vi "Save_to_Project.vi"(8 "error in (no error)":errorcluster, 9 "index":string, 10 "buildObject":T1, 11 "Class in":refnum<class "IB_DistPart.lvclass">) -> (0 "error out":errorcluster, 2 "buildObject out":T1, 3 "Class out":refnum<class "IB_DistPart.lvclass">, 5 "saved?":bool)   [LabVIEW 2020, in "IB_DistPart.lvclass"]
uses:
  <vilib>/AppBuilder/IB_Classes/DistPart/IB_DistPart.lvclass
  <vilib>/AppBuilder/IB_Classes/DistPart/IB_DistPart.lvclass/IB_DistPart.ctl
  <vilib>/AppBuilder/IB_RW_Project/IB_RW_Project_PropBag_Action.ctl
  <vilib>/AppBuilder/IB_Classes/SoftDependency/IB_SoftDependency.lvclass
  <resource>/Framework/Providers/API/ItemRef.ctl
  <vilib>/AppBuilder/IB_RW_Project/IB_RW_Project_DistPart_Data.ctl
panel:
  in  "DistPart":T2
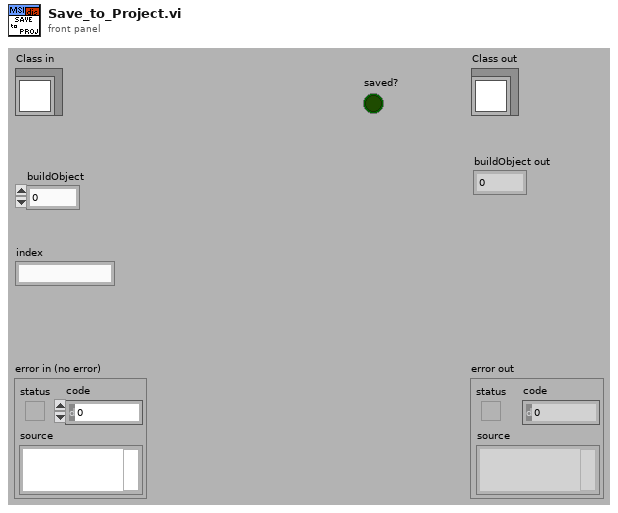
[diagram p1: front panel]
types:
  T1 = typedef "ItemRef.ctl" = u64
  T2 = typedef "IB_RW_Project_DistPart_Data.ctl" = cluster{"ProductId":string, "FlavorId":string, "ProdName":string, "UpgradeCode":string}
  T3 = typedef "IB_RW_Project_PropBag_Action.ctl" = enum16{"read", "write", "clear", "readPrevious", "writePrevious", "clearPrevious"}
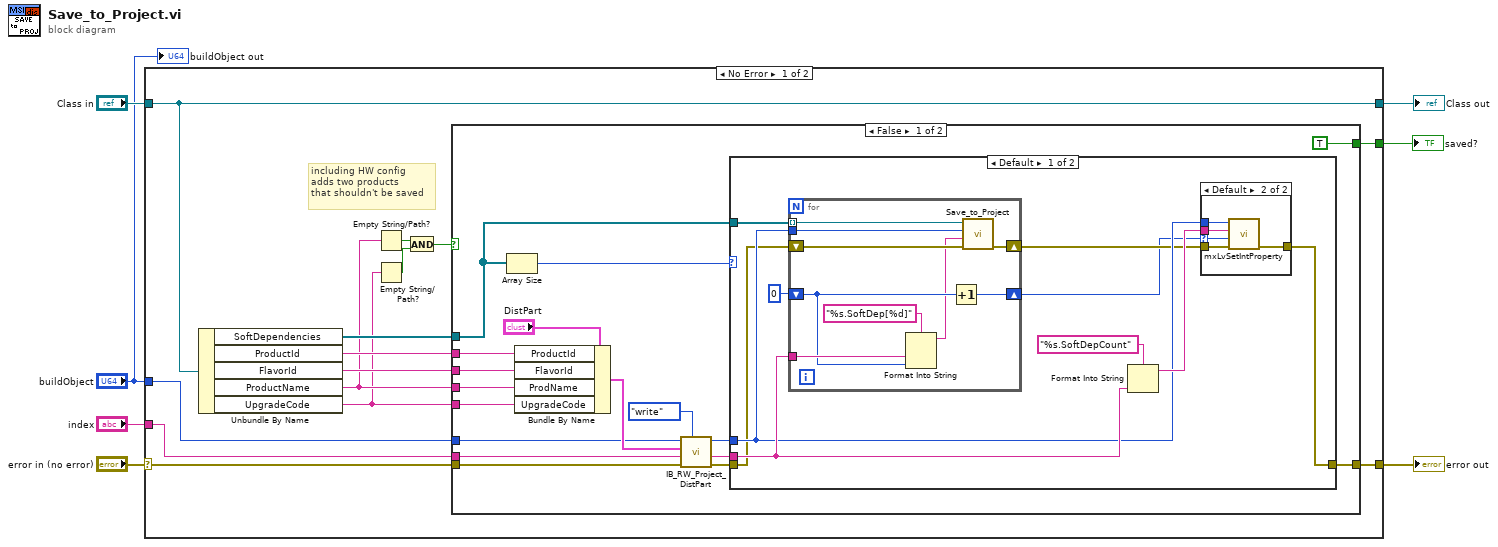
[diagram p0: block diagram]
diagram:
  n1 = case shown="No Error" "error in (no error)" {
    selector: "error in (no error)" -> [w18 w67]
    tunnel: [w15 w67] -> w6
    tunnel: [w19 w66] -> w4
    tunnel: "Class in" -> [w19 w66]
    tunnel: "buildObject" -> [w17 _]
    tunnel: "index" -> [w16 _]
    tunnel: [w8 _] -> w1
    frame No Error {
      # "including HW config\nadds two products\nthat shouldn't be saved"
      n2 = Unbundle By Name(w19) -> ("SoftDependencies"=w14:refnum<class "IB_SoftDependency.lvclass">[], "ProductId"=w21:string, "FlavorId"=w20:string, "ProductName"=w13:string, "UpgradeCode"=w12:string)
      n3 = Empty String/Path?(string/path=w13) -> (empty?=w11:bool)
      n4 = Empty String/Path?(string/path=w12) -> (empty?=w10:bool)
      n5 = And(x=w11, y=w10) -> (x .and. y?=w9:bool)
      n6 = case shown="False" w9 {
        tunnel: w21 -> [w38 _]
        tunnel: w20 -> [w37 _]
        tunnel: w13 -> [w36 _]
        tunnel: w12 -> [w35 _]
        tunnel: w18 -> [w32 w65]
        tunnel: w17 -> [w31 _]
        tunnel: w16 -> [w30 _]
        tunnel: [w27 w65] -> w15
        tunnel: w14 -> [w25 _]
        tunnel: [TRUE _] -> w8
        frame False {
          n7 = Array Size(array=w25) -> (size(s)=w26:i32)
          n8 = Bundle By Name(cluster="DistPart", "ProductId"=w38, "FlavorId"=w37, "ProdName"=w36, "UpgradeCode"=w35) -> (w33:T2)
          n9 = call <vilib>:"IB_RW_Project_DistPart.vi"("action"=IB_RW_Project_PropBag_Action."write", "error in (no error)"=w32, "index in"=w30, "DistParts"=w33, "buildObject"=w31) -> ("error out"=w28:errorcluster, "index out"=w23:string, "buildObject out"=w24:T1)  [unwired: 4 out]
          n10 = case shown="Default" w26 {
            tunnel: w24 -> [w44 _]
            tunnel: w25 -> [w46 _]
            tunnel: w28 -> [w40 w64]
            tunnel: [w42 w64] -> w27
            tunnel: w23 -> [w45 _]
            frame Default {
              n11 = for {
                tunnel: w46 -> [w57] mode=indexing
                tunnel: w44 -> [w62]
                tunnel: w45 -> [w63]
                shift-right: [w61] -> w43
                shift-left: w40 -> [w60]
                shift-right: [w58] -> w39
                shift-left: 0 -> [w59]
                n12 = Format Into String(format string="%s.SoftDep[%d]", w63, w59) -> (resulting string=w55:string)  [unwired: 2 in, 1 out]
                n13 = Increment(x=w59) -> (x+1=w58:i32)
                n14 = call <vilib>:"Save_to_Project.vi"("error in (no error)"=w60, "index in"=w55, "buildObject"=w62, "IB_SoftDependency in"=w57) -> ("error out"=w61:errorcluster)  [unwired: 7 out]
              }
              n15 = Format Into String(format string="%s.SoftDepCount", w45) -> (resulting string=w47:string)  [unwired: 2 in, 1 out]
              n16 = case shown="Default" w39 {
                selector: w39 -> [_ w50]
                tunnel: w47 -> [_ w54]
                tunnel: w44 -> [_ w53]
                tunnel: w43 -> [w49 w52]
                tunnel: [w49 w51] -> w42
                frame 0 {
                }
                frame Default {
                  n17 = call <resource>:"mxLvSetIntProperty.vi"("error in"=w52, "Value (0)"=w50, "Tag"=w54, "Item"=w53) -> ("error out"=w51:errorcluster)  [unwired: 1 in, 6 out]
                }
              }
            }
            frame 0 {
            }
          }
        }
        frame True {
        }
      }
    }
    frame Error {
    }
  }
  "error out" <- w6
  "Class out" <- w4
  "saved?" <- w1
  "buildObject out" <- "buildObject"
